vi "myRIO v1.0 Get Scaling Constant Accelerometer.vi"(8 "error in (no error)":errorcluster) -> (0 "error out":errorcluster, 2 "LSB Weight (g-force/bit)":dbl)   [LabVIEW 2021]
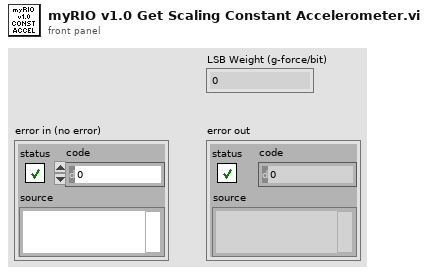
[diagram p1: front panel]
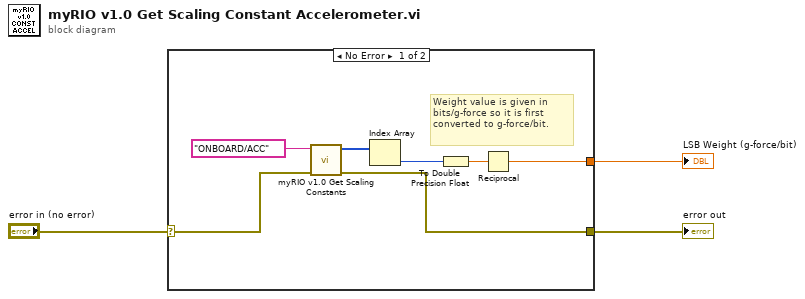
[diagram p0: block diagram]
diagram:
  n1 = case shown="No Error" "error in (no error)" {
    selector: "error in (no error)" -> [w5 w11]
    tunnel: [w4 w11] -> w3
    tunnel: [w9 _] -> w1
    frame No Error {
      # "Weight value is given in bits/g-force so it is first converted to g-force/bit."
      n2 = call <vilib>:"myRIO v1.0 Get Scaling Constants.vi"("error in (no error)"=w5, "Channel Name"="ONBOARD/ACC") -> ("error out"=w4:errorcluster, "Channel Scaling"=w6:u32[])  [unwired: 8 in]
      n3 = Index Array(array=w6) -> (element=w8:u32)  [unwired: 1 in]
      n4 = To Double Precision Float(number=w8) -> (double precision float=w10:dbl)
      n5 = Reciprocal(x=w10) -> (1/x=w9:dbl)
    }
    frame Error {
      # "There is an incoming error so there it nothing to do."
    }
  }
  "error out" <- w3
  "LSB Weight (g-force/bit)" <- w1
